vi "Write Action VI Properties.vi"(8 "error in (no error)":errorcluster, 10 "Path":T1, 11 "ActionVI in":refnum<class "ActionVI.lvclass">) -> (0 "error out":errorcluster, 3 "ActionVI out":refnum<class "ActionVI.lvclass">)   [LabVIEW 2015, in "ActionVI.lvclass"]
uses:
  ActionVI.lvclass
  XML Controls/Path Cluster.ctl
  ActionVI.lvclass/ActionVI.ctl
  VeriStand Custom Device XML Parser.lvlib
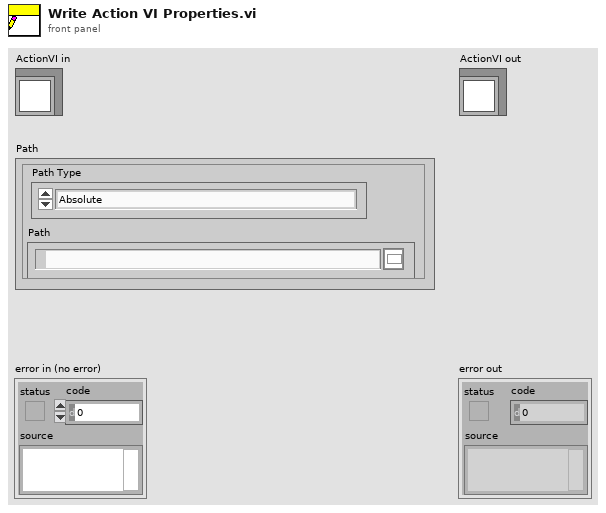
[diagram p1: front panel]
types:
  T1 = typedef "VeriStand Custom Device XML Parser.lvlib/Path Cluster.ctl" = cluster{"Path":path, "Path Type":enum16{"Absolute", "To Base", "To Common Doc Dir", "To Application Data Dir"}}
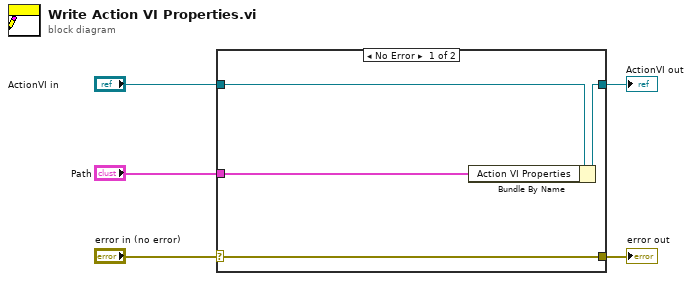
[diagram p0: block diagram]
diagram:
  n1 = case shown="No Error" "error in (no error)" {
    selector: "error in (no error)" -> [w9 w10]
    tunnel: [w9 w10] -> w4
    tunnel: [w7 w11] -> w2
    tunnel: "ActionVI in" -> [w8 w11]
    tunnel: "Path" -> [w6 _]
    frame No Error {
      n2 = Bundle By Name(cluster=w8, "Action VI Properties"=w6) -> (w7:refnum<class "ActionVI.lvclass">)
    }
    frame Error {
    }
  }
  "error out" <- w4
  "ActionVI out" <- w2
